vi "RouteGuideUnaryRouteGuideTest.vi"() -> ()   [LabVIEW 2019]
uses:
  gRPC_ATS/TestUtility/utility.llb/array of error description.ctl
  gRPC_ATS/TestUtility/utility.llb/error description.ctl
  gRPC_ATS/TestUtility/utility.llb/error type.ctl
panel:
  out "Array of Error Description":T1
  out "Pass?":bool
  in  "Client VI Path":path
  in  "Server VI path":path
  in  "error in (no error)":errorcluster
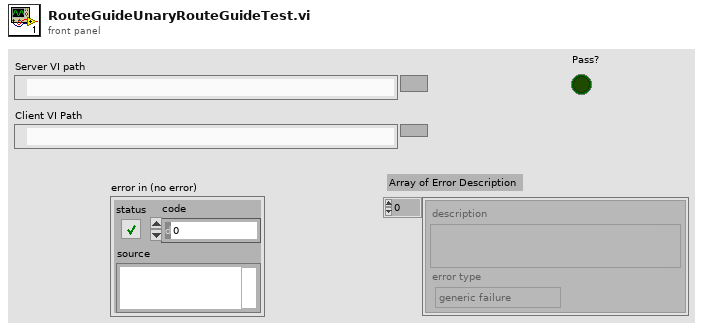
[diagram p1: front panel]
types:
  T1 = typedef "array of error description.ctl" = T2[]
  T2 = typedef "error description.ctl" = cluster{"description":string, "error type":T3}
  T3 = typedef "error type.ctl" = enum32{"generic failure", "boundary case", "precision", "expected error"}
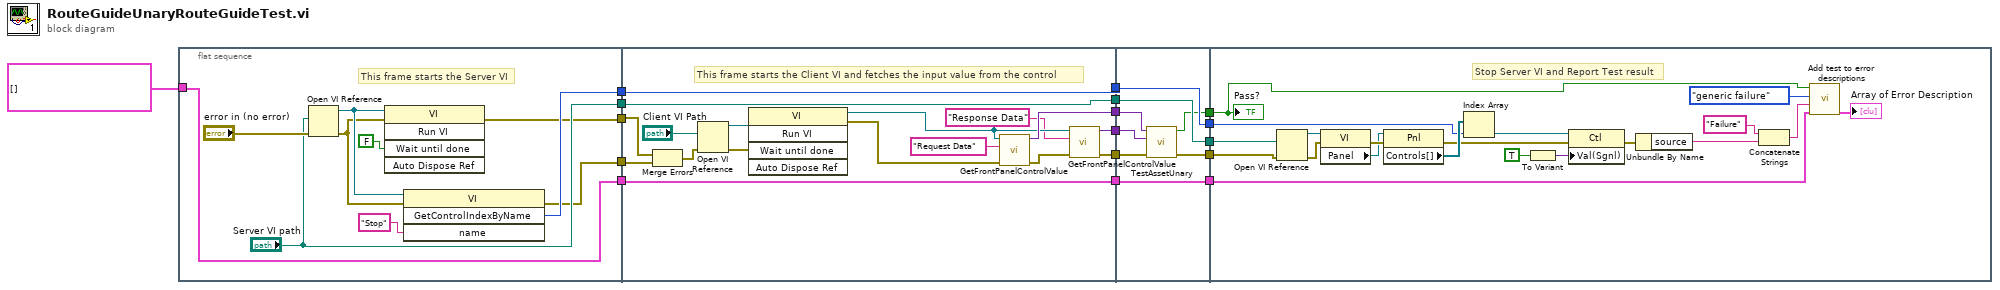
[diagram p0: block diagram]
diagram:
  n1 = flat-sequence {
    tunnel: [w24] -> w17
    tunnel: ["Server VI path"] -> w16
    tunnel: T1 [] ("error descriptions in") -> [w21]
    tunnel: [w21] -> w15
    tunnel: [w19] -> w2
    tunnel: [w18] -> w1
    tunnel: w17 -> [w40]
    tunnel: w16 -> [w41]
    tunnel: [w41] -> w14
    tunnel: [w40] -> w13
    tunnel: w15 -> [w39]
    tunnel: [w39] -> w12
    tunnel: [w31] -> w6
    tunnel: [w36] -> w5
    tunnel: [w32] -> w4
    tunnel: w2 -> [w30]
    tunnel: w1 -> [w29]
    tunnel: w14 -> [w50]
    tunnel: [w50] -> w11
    tunnel: w13 -> [w52]
    tunnel: [w52] -> w10
    tunnel: [w48] -> w9
    tunnel: w12 -> [w51]
    tunnel: [w51] -> w8
    tunnel: w6 -> [w49]
    tunnel: w5 -> [w45]
    tunnel: w4 -> [w46]
    tunnel: [w47] -> w3
    tunnel: w11 -> [w72]
    tunnel: w10 -> [w67]
    tunnel: w9 -> [w62]
    tunnel: w8 -> [w56]
    tunnel: w3 -> [w53]
    frame #0 {
      # "This frame starts the Server VI"
      n2 = Open VI Reference(vi path="Server VI path", error in (no error)="error in (no error)") -> (vi reference=w23:refnum<vi>, error out=w20:errorcluster)  [unwired: 4 in]
      n3 = invoke class="VI" method="Run VI"(reference=w23, error in=w20, "Wait until done"=FALSE ("Wait Until Done")) -> (error out=w19:errorcluster)  [unwired: 2 in, 4 out]
      n4 = invoke class="VI" method="GetControlIndexByName"(reference=w23, error in=w20, "name"="Stop" ("Control Name")) -> (error out=w18:errorcluster, "GetControlIndexByName"=w24:i32)  [unwired: 1 in, 2 out]
    }
    frame #1 {
      # "This frame starts the Client VI and fetches the input value from the control"
      n5 = Merge Errors(w30, w29) -> (w28:errorcluster)
      n6 = Open VI Reference(vi path="Client VI Path", error in (no error)=w28) -> (vi reference=w43:refnum<vi>, error out=w42:errorcluster)  [unwired: 4 in]
      n7 = invoke class="VI" method="Run VI"(reference=w43, error in=w42) -> (reference out=w35:refnum<vi>, error out=w38:errorcluster)  [unwired: 3 in, 3 out]
      n8 = call "GetFrontPanelControlValue.vi"("error in"=w38, "Control Name"="Request Data", "reference"=w35) -> ("error out"=w33:errorcluster, "Value"=w36:variant)  [unwired: 7 in]
      n9 = call "GetFrontPanelControlValue.vi"("error in"=w33, "Control Name"="Response Data", "reference"=w35) -> ("error out"=w31:errorcluster, "Value"=w32:variant)  [unwired: 7 in]
    }
    frame #2 {
      n10 = call "TestAssetUnary.vi"("Test Input"=w45, "Test Output"=w46, "error in"=w49) -> ("Pass?"=w48:bool, "error out"=w47:errorcluster)  [unwired: 6 in]
    }
    frame #3 {
      # "Stop Server VI and Report Test result"
      n11 = Open VI Reference(vi path=w72, error in (no error)=w53) -> (vi reference=w71:refnum<vi>, error out=w55:errorcluster)  [unwired: 4 in]
      n12 = property class="VI"(reference=w71, error in=w55) -> (error out=w70:errorcluster, "Panel"=w69:refnum<vi>)  [unwired: 1 out]
      n13 = property class="Pnl"(reference=w69, error in=w70) -> (error out=w54:errorcluster, "Controls[]"=w68:refnum<vi>[])  [unwired: 1 out]
      n14 = Index Array(array=w68, index=w67) -> (element=w66:refnum<vi>)
      n15 = To Variant(anything=TRUE) -> (Variant=w65:variant)
      n16 = property class="Ctl"(reference=w66, error in=w54, "Val(Sgnl)"=w65) -> (error out=w59:errorcluster)  [unwired: 1 out]
      n17 = Unbundle By Name(w59) -> ("source"=w58:string)
      n18 = Concatenate Strings("Failure" ("string"), w58) -> (w60:string)
      n19 = call "Add test to error descriptions.vi"("error descriptions in"=w56, "error string"=w60, "error type"=error_type."generic failure", "pass"=w62) -> ("error description out"=→"Array of Error Description":T1)  [unwired: 3 in]
      "Pass?" <- w62
    }
  }
